vi "DMM Wrapper.vi"(7 "Control":T1=enum."Close", 8 "error in":errorcluster, 10 "Channel Index":i32, 11 "Setting":T2={"Resolution (Digits)"=5.5, "Current Source (Amps)"=0.001, "Range"=2.0, "Measurement Type"=enum."DC Volts"} {"Range" format="%.2p"; "Current Source (Amps)" items=["1uA"=1e-06, "10uA"=1e-05, "100uA"=0.0001, "1mA"=0.001]; "Resolution (Digits)" items=["3 1/2"=3.5, "4 1/2"=4.5, "5 1/2"=5.5, "6 1/2"=6.5, "7 1/2"=7.5]}) -> (0 "error out":errorcluster, 3 "Measurement":dbl=nan)   [LabVIEW 2021]
uses:
  Controls/DMM States.ctl
  Load INI/Controls/Instruments_Data.ctl
  Load INI/Controls/MUX_Data.ctl
  Load INI/Controls/DMM_Data.ctl
  <vilib>/numeric/Random Number (Range) DBL.vi
  <instrlib>/niDMM/nidmm.llb/niDMM Configure Measurement Digits.vi
  <instrlib>/niSwitch/niSwitch.llb/niSwitch Connect Channels (Multiple).vi
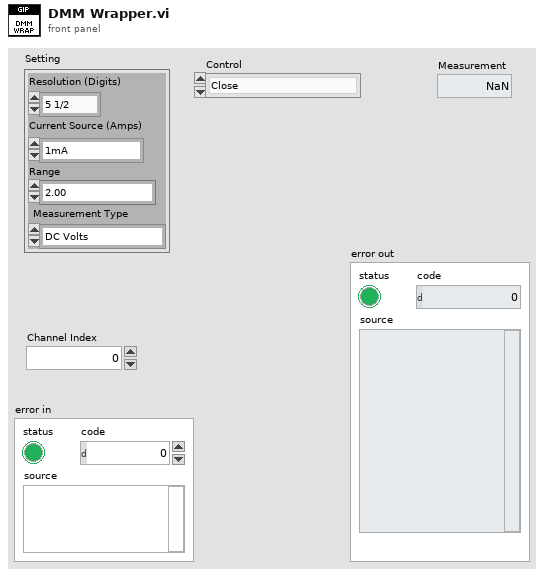
[diagram p1: front panel]
types:
  T1 = typedef "DMM States.ctl" = enum16{"Init", "Get Switch Ref", "Config", "Read", "Close"}
  T2 = cluster{"Resolution (Digits)":dbl, "Current Source (Amps)":dbl, "Range":dbl, "Measurement Type":enum16{"DC Volts", "AC Volts", "DC Current", "AC Current", "2-wire Resistance", "4-wire Resistance", "Diode", "Frequency", "Period", "AC Volts DC Coupled", "Capacitance", "Inductance", "Temperature"}}
  T3 = typedef "Instruments_Data.ctl" = cluster{"Alias":string, "Resource ":string}
  T4 = cluster{"DMM ref":refnum<k15>, "SW Refs":refnum<k15>[]}
  T5 = typedef "MUX_Data.ctl" = cluster{"Alias":string, "Topology":string}
  T6 = typedef "DMM_Data.ctl" = cluster{"Alias":string, "MUX":string, "Route":string}
  T7 = enum16{"DC Volts", "AC Volts", "DC Current", "AC Current", "2-wire Resistance", "4-wire Resistance", "Diode", "Frequency", "Period", "AC Volts DC Coupled", "Capacitance", "Inductance", "Temperature"}
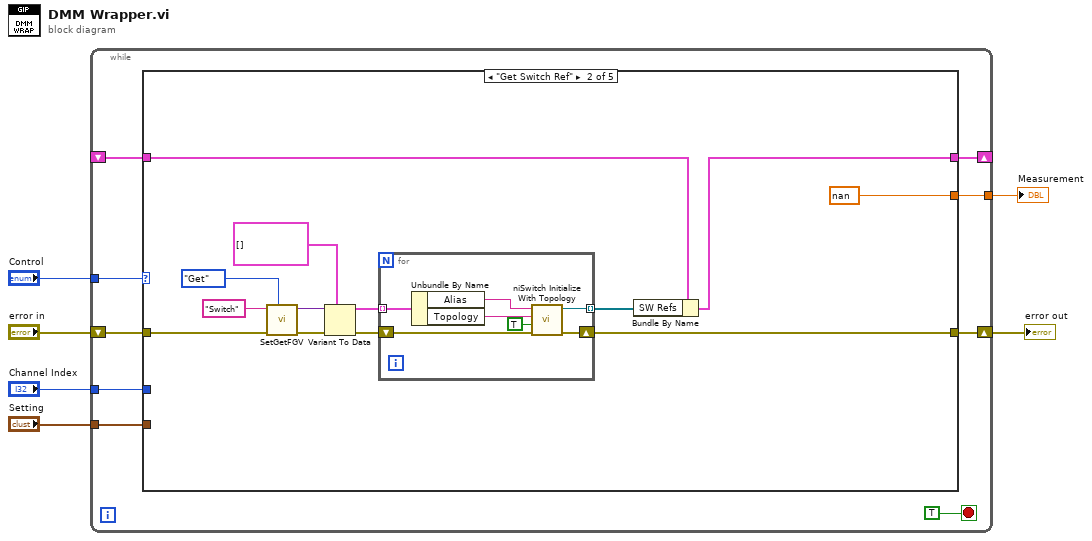
[diagram p0: block diagram]
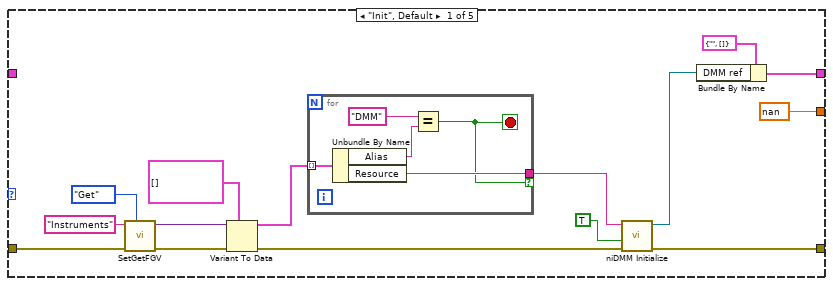
[diagram p2: hidden frame]
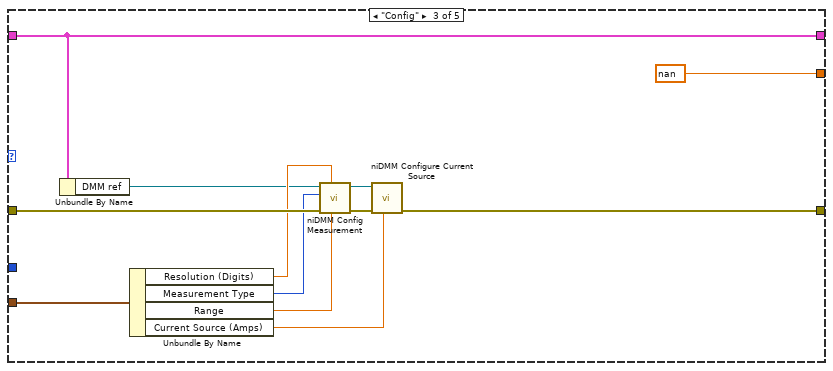
[diagram p3: hidden frame]
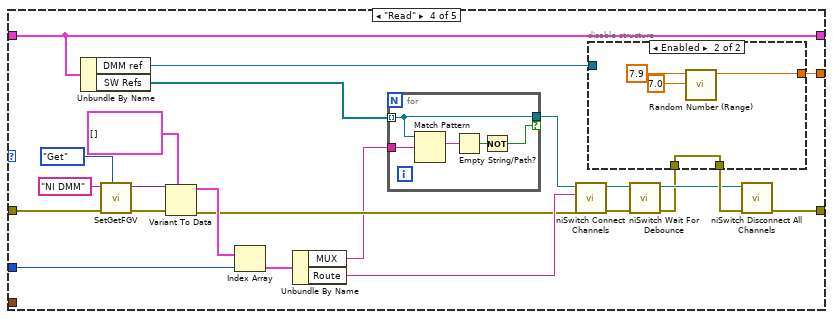
[diagram p4: hidden frame]
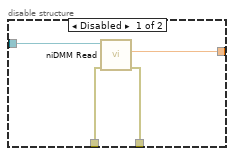
[diagram p5: hidden frame]
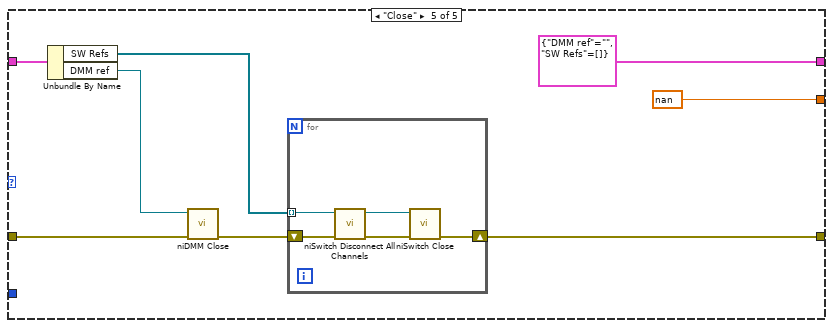
[diagram p6: hidden frame]
diagram:
  n1 = while {
    tunnel: "Setting" -> [w13]
    tunnel: [w12] -> w5
    tunnel: "Control" -> [w11]
    shift-right: [w14] -> w1
    shift-left: "error in" -> [w15]
    shift-right: [w9] -> _
    shift-left: _ -> [w8]
    tunnel: "Channel Index" -> [w7]
    stop <- TRUE stop-if-true
    n2 = case shown="\"Get Switch Ref\"" w11 {
      tunnel: w15 -> [w24 w40 w66 w87 w107]
      tunnel: [w27 w39 w57 w89 w106] -> w14
      tunnel: [w29 w37 w58 w90 T4 {"DMM ref"="", "SW Refs"=[]}] -> w9
      tunnel: w8 -> [_ w38 w58 w90 w108]
      tunnel: w13 -> [_ _ w64 _ _]
      tunnel: [nan nan nan w88 nan] -> w12
      tunnel: w7 -> [_ _ _ w86 _]
      frame "Init", Default {
        n3 = call "SetGetFGV.vi"("Method (Get)"=enum16{"Get", "Set"}."Get", "error in"=w24, "FGVname"="Instruments" ("Name")) -> ("error out"=w23:errorcluster, "Data out"=w19:variant)  [unwired: 7 in]
        n4 = Variant To Data(error in=w23, type=T3[] [], Variant=w19) -> (data=w17:T3[], error out=w20:errorcluster)
        n5 = for {
          tunnel: w17 -> [w35] mode=indexing
          tunnel: [w32] -> w16 if=w31
          stop <- w31 stop-if-true
          n6 = Unbundle By Name(w35) -> ("Alias"=w34:string, "Resource"=w32:string)
          n7 = Equal?(x="DMM" ("Name"), y=w34) -> (x = y?=w31:bool)
        }
        n8 = call <instrlib>:"niDMM Initialize.vi"("error in (no error)"=w20, "Reset"=TRUE ("ID Query? (T: Yes)"), "Instrument Descriptor"=w16) -> ("error out"=w27:errorcluster, "instrument handle out"=w25:refnum<k15>)  [unwired: 1 in, 6 out]
        n9 = Bundle By Name(cluster=T4 {"DMM ref"="", "SW Refs"=[]}, "DMM ref"=w25) -> (w29:T4)
      }
      frame "Get Switch Ref" {
        n10 = call "SetGetFGV.vi"("Method (Get)"=enum16{"Get", "Set"}."Get", "error in"=w40, "FGVname"="Switch" ("Name")) -> ("error out"=w48:errorcluster, "Data out"=w47:variant)  [unwired: 7 in]
        n11 = Variant To Data(error in=w48, type=T5[] [], Variant=w47) -> (data=w46:T5[], error out=w45:errorcluster)
        n12 = for {
          tunnel: w46 -> [w54] mode=indexing
          tunnel: [w51] -> w44 mode=indexing
          shift-right: [w50] -> w39
          shift-left: w45 -> [w55]
          n13 = Unbundle By Name(w54) -> ("Alias"=w53:string, "Topology"=w52:string)
          n14 = call <instrlib>:"niSwitch Initialize With Topology.vi"("error in (no error)"=w55, "reset device (boolean value)"=TRUE, "topology name"=w52, "resource name"=w53) -> ("error out"=w50:errorcluster, "instrument handle out"=w51:refnum<k15>)  [unwired: 6 in]
        }
        n15 = Bundle By Name(cluster=w38, "SW Refs"=w44) -> (w37:T4)
      }
      frame "Config" {
        n16 = Unbundle By Name(w58) -> ("DMM ref"=w56:refnum<k15>)
        n17 = Unbundle By Name(w64) -> ("Resolution (Digits)"=w60:dbl, "Measurement Type"=w63:T7, "Range"=w59:dbl, "Current Source (Amps)"=w61:dbl)
        n18 = call-poly <instrlib>:"niDMM Config Measurement.vi"("Range"=w59, "Resolution in Digits"=w60, "error in (no error)"=w66, "Function"=w63, "instrument handle"=w56) -> ("error out"=w67:errorcluster, "instrument handle out"=w65:refnum<k15>)  [unwired: 5 out]
        n19 = call <instrlib>:"niDMM Configure Current Source.vi"("Current Source"=w61, "error in (no error)"=w67, "instrument handle"=w65) -> ("error out"=w57:errorcluster)  [unwired: 1 in, 7 out]
      }
      frame "Read" {
        n20 = Unbundle By Name(w90) -> ("DMM ref"=w68:refnum<k15>, "SW Refs"=w71:refnum<k15>[])
        n21 = call "SetGetFGV.vi"("Method (Get)"=enum16{"Get", "Set"}."Get", "error in"=w87, "FGVname"="NI DMM" ("Name")) -> ("error out"=w81:errorcluster, "Data out"=w80:variant)  [unwired: 7 in]
        n22 = Variant To Data(error in=w81, type=T6[] [], Variant=w80) -> (data=w74:T6[], error out=w72:errorcluster)
        n23 = Index Array(array=w74, index=w86) -> (element=w75:T6)
        n24 = Unbundle By Name(w75) -> ("MUX"=w70:string, "Route"=w77:string)
        n25 = for {
          tunnel: w71 -> [w100] mode=indexing
          tunnel: w70 -> [w103]
          tunnel: [w100] -> w69 if=w99
          n26 = Match Pattern(string=w100, regular expression=w103) -> (match substring=w102:string)  [unwired: 1 in, 3 out]
          n27 = Empty String/Path?(string/path=w102) -> (empty?=w101:bool)
          n28 = Not(x=w101) -> (.not. x?=w99:bool)
        }
        n29 = call-poly <instrlib>:"niSwitch Connect Channels.vi"("error in (no error)"=w72, "connection list"=w77, "instrument handle"=w69) -> ("error out"=w73:errorcluster, "instrument handle out"=w83:refnum<k15>)  [unwired: 7 in]
        n30 = call <instrlib>:"niSwitch Wait For Debounce.vi"("error in (no error)"=w73, "instrument handle"=w83) -> ("error out"=w78:errorcluster, "instrument handle out"=w84:refnum<k15>)  [unwired: 1 in, 7 out]
        n31 = disable-structure shown="Enabled" {
          disable-tunnel: [w94 w95] -> w88
          disable-tunnel: [w93 w96] -> w85
          disable-tunnel: w78 -> [w92 w96]
          disable-tunnel: w68 -> [w91 _]
          frame Disabled {
            n32 = call <instrlib>:"niDMM Read.vi"("error in (no error)"=w92, "instrument handle"=w91) -> ("error out"=w93:errorcluster, "Measurement"=w94:dbl)  [unwired: 1 in, 7 out]
          }
          frame Enabled {
            n33 = call-poly <vilib>:"Random Number (Range).vi"("lower bound (0)"=7.0, "upper bound (100)"=7.9) -> ("number"=w95:dbl)  [unwired: 9 in]
          }
        }
        n34 = call <instrlib>:"niSwitch Disconnect All Channels.vi"("error in (no error)"=w85, "instrument handle"=w84) -> ("error out"=w89:errorcluster)  [unwired: 8 in, 1 out]
      }
      frame "Close" {
        n35 = Unbundle By Name(w108) -> ("SW Refs"=w110:refnum<k15>[], "DMM ref"=w104:refnum<k15>)
        n36 = call <instrlib>:"niDMM Close.vi"("error in (no error)"=w107, "instrument handle"=w104) -> ("error out"=w109:errorcluster)  [unwired: 9 in]
        n37 = for {
          tunnel: w110 -> [w112] mode=indexing
          shift-right: [w116] -> w106
          shift-left: w109 -> [w113]
          n38 = call <instrlib>:"niSwitch Disconnect All Channels.vi"("error in (no error)"=w113, "instrument handle"=w112) -> ("error out"=w115:errorcluster, "instrument handle out"=w114:refnum<k15>)  [unwired: 8 in]
          n39 = call <instrlib>:"niSwitch Close.vi"("error in (no error)"=w115, "instrument handle"=w114) -> ("error out"=w116:errorcluster)  [unwired: 9 in]
        }
      }
    }
  }
  "Measurement" <- w5
  "error out" <- w1
